vi "NI VeriStand - Send Message To Driver VI.vi"(8 "error in (no error)":errorcluster, 9 "Timeout (ms)":i32, 10 "Data":string, 11 "Device Ref in":T1 format="%.0x") -> (0 "error out":errorcluster, 1 "timed out?":bool, 2 "Response Data":string, 3 "Device Ref out":T1 format="%.0x")   [LabVIEW 2020, in "Custom Device API.lvlib"]
uses:
  <vilib>/NI VeriStand/Custom Device API/Custom Device API.lvlib
  <vilib>/NI VeriStand/Custom Device API/Custom Device Item Ref.ctl
  60daa420-b786-4861-a2f1-3618a5dcbfd2.vi
  <vilib>/NI VeriStand/Custom Device API/Custom Device Offline Path.vi
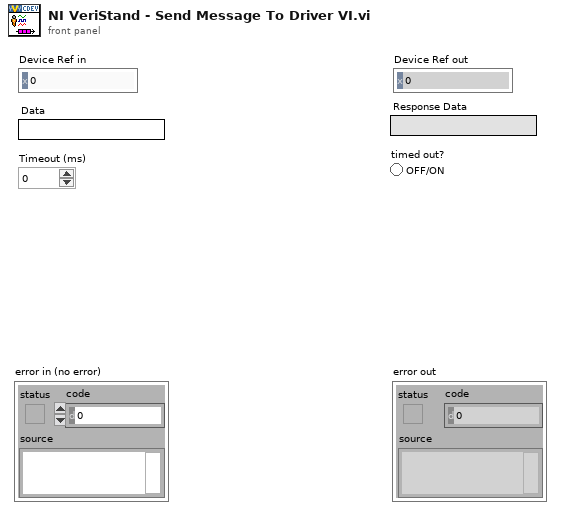
[diagram p1: front panel]
types:
  T1 = typedef "Custom Device API.lvlib/Custom Device Item Ref.ctl" = u64
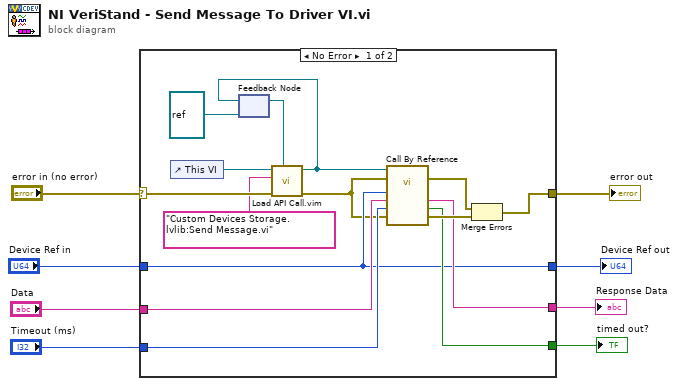
[diagram p0: block diagram]
diagram:
  n1 = case shown="No Error" "error in (no error)" {
    selector: "error in (no error)" -> [w14 w25]
    tunnel: [w22 w25] -> w8
    tunnel: "Device Ref in" -> [w17 w24]
    tunnel: "Data" -> [w21 _]
    tunnel: "Timeout (ms)" -> [w20 _]
    tunnel: [w19 _] -> w4
    tunnel: [w18 _] -> w3
    tunnel: [w17 w24] -> w1
    frame No Error {
      n2 = control-ref of="This VI"() -> (w15:refnum<vi>)
      n3 = feedback #1(refnum<vi> refnum ("type specifier VI Refnum (for type only)")) -> (w16:refnum<vi>)
      n4 = call "Load API Call.vim"("VI reference in"=w16, "error in (no error)"=w14, "VI qualified name"="Custom Devices Storage.lvlib:Send Message.vi", "Caller VI ref"=w15) -> ("error out"=w12:errorcluster, "VI reference"=w13:refnum<vi>)  [unwired: 6 in]
      n5 = feedback-in #1(w13) -> ()
      n6 = call-by-ref "?"(reference=w13, error in=w12, 8:"error in (no error)"=w12, "Timeout (ms)"=w20, "Data"=w21, "Dev Ref in"=w17) -> (error out=w9:errorcluster, 0:"error out"=w23:errorcluster, "timed out?"=w18:bool, "Response Data"=w19:string)  [unwired: 4 in, 2 out]
      n7 = Merge Errors(w9, w23) -> (w22:errorcluster)
    }
    frame Error {
    }
  }
  "Device Ref out" <- w1
  "error out" <- w8
  "Response Data" <- w4
  "timed out?" <- w3
